vi "Formula_Node_Ejercicio.vi"() -> ()   [LabVIEW 2016]
panel:
  out "XY Graph":cluster{dbl[], dbl[]}(graph)
  out "output variable 2":dbl
  out "output variable":dbl
  out "Waveform Graph":dbl[](graph)
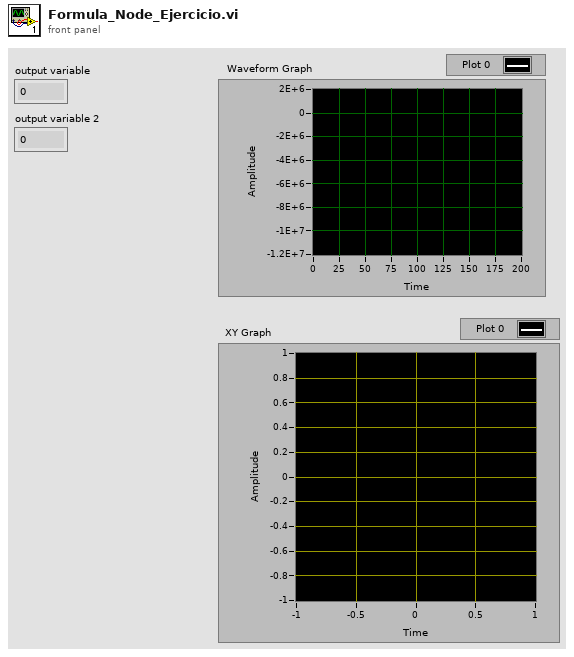
[diagram p1: front panel]
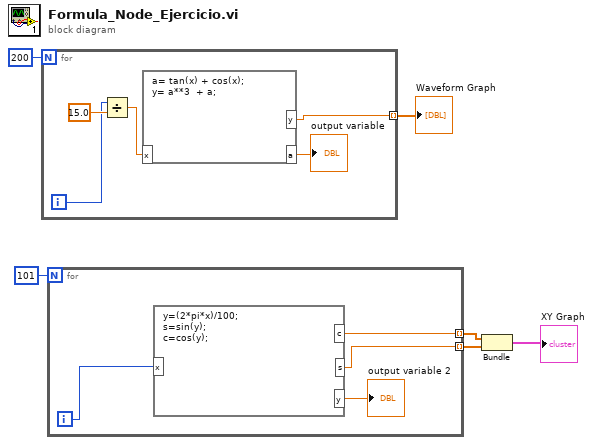
[diagram p0: block diagram]
diagram:
  n1 = for {
    N: 200 -> [_]
    tunnel: [w8] -> w5 mode=indexing
    i -> [w10]
    n2 = Divide(x=w10, y=15.0) -> (x/y=w9:dbl)
    n3 = formula code="a= tan(x) + cos(x);\ny= a**3  + a;"("x"=w9) -> ("y"=w8:dbl, "a"=→"output variable":dbl)
  }
  "Waveform Graph" <- w5
  n4 = for {
    N: 101 -> [_]
    tunnel: [w13] -> w3 mode=indexing
    tunnel: [w12] -> w2 mode=indexing
    i -> [w15]
    n5 = formula code="y=(2*pi*x)/100;\ns=sin(y);\nc=cos(y);"("x"=w15) -> ("s"=w12:dbl, "c"=w13:dbl, "y"=→"output variable 2":dbl)
  }
  n6 = Bundle(w3, w2) -> (→"XY Graph":cluster{dbl[], dbl[]})  [unwired: 1 in]
